vi "Initialize-process-notifiers.vi"(8 "error in (no error)":errorcluster, 11 "Data ref. in":refnum<data-value>) -> (0 "error out":errorcluster, 3 "Data ref.":refnum<data-value>)   [LabVIEW 2013, in "CameraVision.lvlib" / "CV-Main.lvclass"]
uses:
  CV-Main.lvclass
  Buffers/Storage-buffer.ctl
  <vilib>/vision/Image Controls.llb/IMAQ Image.ctl
  Temperature/Temperature-characteristics.ctl
  Analysis/Characteristics-cluster.ctl
  Acquisition/Acquisition-stats.ctl
  Buffers/Mapping-buffer.ctl
  CV-Main.lvclass/CV-Main.ctl
  Temperature/CV-Temperature.lvclass
  Analysis/CV-Analysis.lvclass
  Acquisition/CV-Acquisition.lvclass
  Buffers/CV-Buffers.lvclass
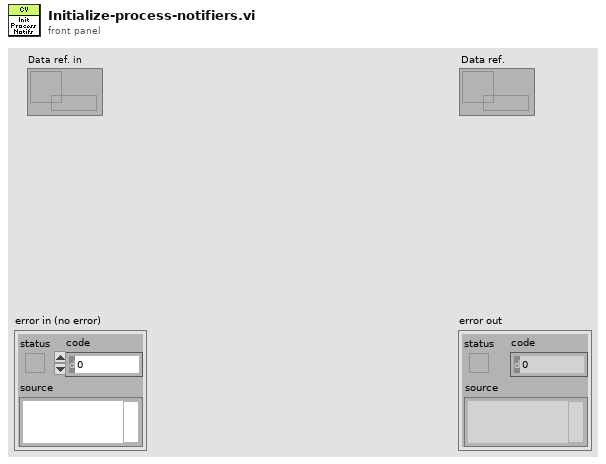
[diagram p1: front panel]
types:
  T1 = typedef "CameraVision.lvlib/CV-Buffers.lvclass/Mapping-buffer.ctl" = cluster{"Time":timestamp, "Index":i32, "Temperature characteristics":T2, "Characteristics":T3[], "Xcoord":sgl, "Ycoord":sgl}
  T2 = typedef "CameraVision.lvlib/CV-Temperature.lvclass/Temperature-characteristics.ctl" = cluster{"Average temperature ":dbl, "Max. temperature":dbl, "Min. temperature":dbl, "Stand. dev. temperature":dbl, "Datapoints":dbl}
  T3 = typedef "CameraVision.lvlib/CV-Analysis.lvclass/Characteristics-cluster.ctl" = cluster{"Average intensity":dbl, "Peak intensity":dbl, "Melt-pool size":dbl, "Melt-pool aspect ratio":dbl, "Melt-pool fragments":dbl, "Centre of mass X":dbl, "Centre of mass Y":dbl, "Orientation":dbl}
  T4 = typedef "CameraVision.lvlib/CV-Acquisition.lvclass/Acquisition-stats.ctl" = cluster{"Index":i32, "Time":timestamp, "Acq duration":dbl, "Process duration":dbl}
  T5 = typedef "CameraVision.lvlib/CV-Buffers.lvclass/Storage-buffer.ctl" = cluster{"Index":i32, "Time":timestamp, "Raw images":T6[], "Corrected images":T6[], "Binary images":T6[], "Temperature characteristics":T2, "Characteristics":T3[], "Temperature field":dbl[][]}
  T6 = typedef "IMAQ Image.ctl" = refnum<image>
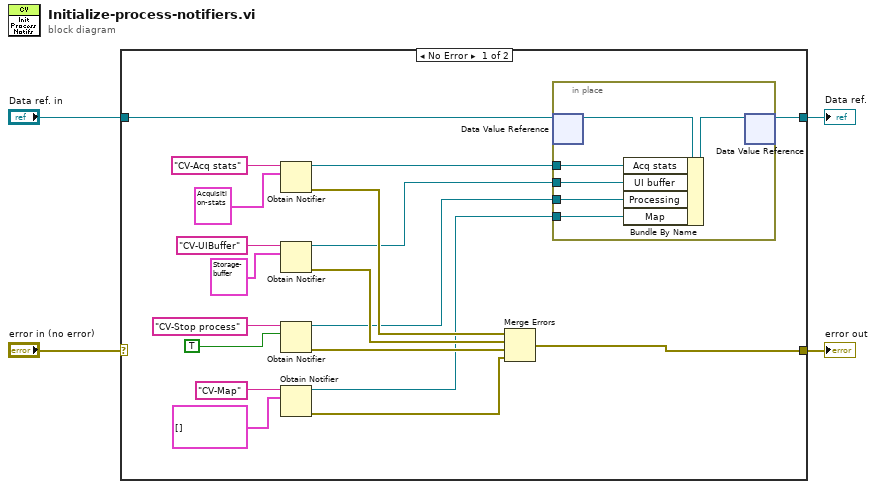
[diagram p0: block diagram]
diagram:
  n1 = case shown="No Error" "error in (no error)" {
    selector: "error in (no error)" -> [_ w31]
    tunnel: [w9 w31] -> w3
    tunnel: "Data ref. in" -> [w23 w30]
    tunnel: [w22 w30] -> w1
    frame No Error {
      n2 = Obtain Notifier(name (unnamed)="CV-Acq stats", notification data type=T4 {"Index"=0, "Time"=timestamp(0 s since 1904-01-01), "Acq duration"=0.0, "Process duration"=0.0} ("Acq. stats")) -> (notifier out=w12:refnum<notifier>, error out=w18:errorcluster)  [unwired: 2 in, 1 out]
      n3 = Obtain Notifier(name (unnamed)="CV-UIBuffer", notification data type=T5 {"Index"=0, "Time"=timestamp(0 s since 1904-01-01), "Raw images"=[], "Corrected images"=[], "Binary images"=[], "Temperature characteristics"={"Average temperature "=0.0, "Max. temperature"=0.0, "Min. temperature"=0.0, "Stand. dev. temperature"=0.0, "Datapoints"=0.0}, "Characteristics"=[], "Temperature field"=[]} ("Storage element")) -> (notifier out=w11:refnum<notifier>, error out=w17:errorcluster)  [unwired: 2 in, 1 out]
      n4 = Obtain Notifier(name (unnamed)="CV-Stop process", notification data type=TRUE) -> (notifier out=w10:refnum<notifier>, error out=w14:errorcluster)  [unwired: 2 in, 1 out]
      n5 = Obtain Notifier(name (unnamed)="CV-Map", notification data type=T1[] []) -> (notifier out=w6:refnum<notifier>, error out=w7:errorcluster)  [unwired: 2 in, 1 out]
      n6 = Merge Errors(w18, w17, w14, w7) -> (w9:errorcluster)
      n7 = in-place {
        in-place-border: w12 -> [w27]
        in-place-border: w11 -> [w26]
        in-place-border: w10 -> [w25]
        in-place-border: w6 -> [w24]
        n8 = in-place-dvr #1(w23) -> (w29:refnum<class "CV-Main.lvclass">)  [unwired: 1 out]
        n9 = Bundle By Name(cluster=w29, "Acq stats"=w27, "UI buffer"=w26, "Processing"=w25, "Map"=w24) -> (w28:refnum<class "CV-Main.lvclass">)
        n10 = in-place-dvr #1(w28) -> (w22:refnum<data-value>)  [unwired: 1 out]
      }
    }
    frame Error {
    }
  }
  "error out" <- w3
  "Data ref." <- w1
